vi "Read (Multiple Points).vi"(0 "VISA resource name":refnum<visa-resource-name>, 1 "Timeout (10000 ms)":i32=10000, 2 "Start Index (1)":i32=1, 3 "End Index(10)":i32=10, 5 "Buffer Name (\"\")":string, 7 "Capture Mode(0: Scan)":i32(ring) items=["Scan", "Trigger"], 9 "Clear Buffer (No)":bool, 11 "error in (no error)":errorcluster, 12 "Buffer Element1 ()":i32(ring) items=["", "Date", "Extra", "Formatted", "Fractional", "Reading", "Relative", "Seconds", "Status", "Time", "Tstamp", "Unit", "CHAN", "Extra Format", "Extra Unit"], 13 "Buffer Element2 ()":i32(ring) items=["", "Date", "Extra", "Formatted", "Fractional", "Reading", "Relative", "Seconds", "Status", "Time", "Tstamp", "Unit", "CHAN", "Extra Form", "Extra Unit"], 14 "Get Full Buffer":bool=TRUE) -> (4 "VISA resource name out":refnum<visa-resource-name>, 6 "Measurements":dbl[](array[numeric]), 15 "error out":errorcluster)   [LabVIEW 2020, in "Keithley DMM6500 DAQ6500 Series.lvlib"]
doc: "Reads and returns multiple measurements from the instrument. Use this VI when you want to take multiple measurements using an immediate trigger. Use the low-level VIs for other triggering options."
uses:
  <instrlib>/Keithley DMM6500 DAQ6500 Series/Keithley DMM6500 DAQ6500 Series.lvlib
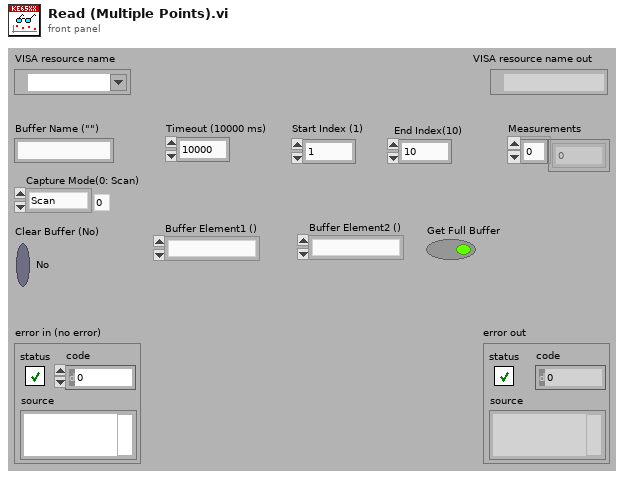
[diagram p1: front panel]
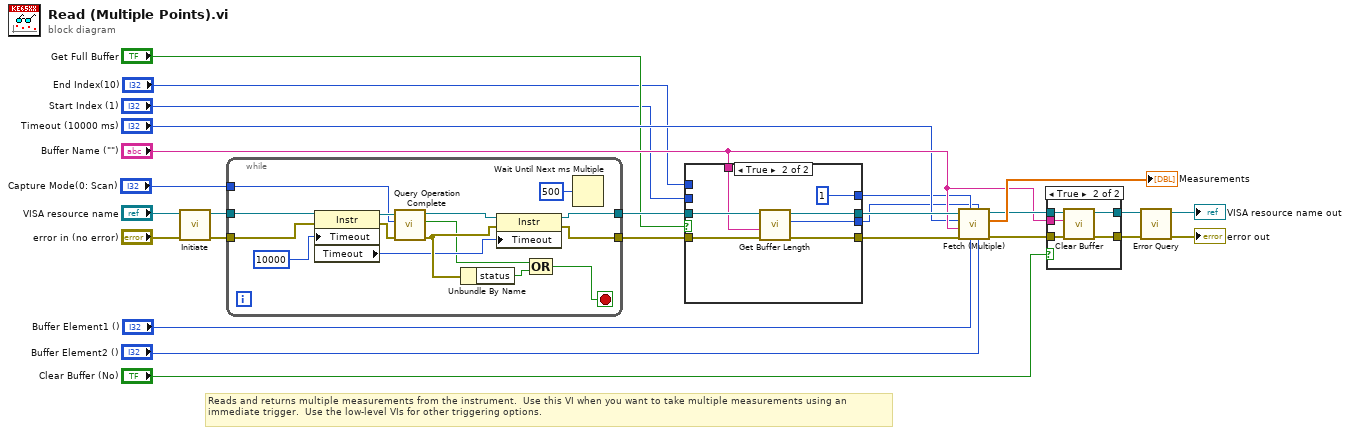
[diagram p0: block diagram]
diagram:
  # "Reads and returns multiple measurements from the instrument.  Use this VI when you want to take multiple measurements using an immediate trigger.  Use the low-level VIs for other triggering options."
  n1 = call <instrlib>:"Initiate.vi"("error in (no error)"="error in (no error)", "VISA resource name"="VISA resource name") -> ("error out"=w19:errorcluster, "VISA resource name out"=w20:refnum<visa-resource-name>)  [unwired: 8 in]
  n2 = while {
    tunnel: w20 -> [w38]
    tunnel: w19 -> [w37]
    tunnel: [w34] -> w16
    tunnel: [w33] -> w15
    tunnel: "Capture Mode(0: Scan)" -> [w27]
    stop <- w40 stop-if-true
    n3 = property on="Property Node" class="Instr"(reference=w38, error in=w37, "Timeout"=u32 10000 ("General Settings:Timeout Value")) -> (reference out=w36:refnum<visa-resource-name>, error out=w35:errorcluster, "Timeout"=w30:u32)
    n4 = call <instrlib>:"Query Operation Complete.vi"("error in (no error)"=w35, "Capture Mode (0: Scan)"=w27, "VISA resource name"=w36) -> ("error out"=w31:errorcluster, "Complete"=w28:bool, "VISA resource name out"=w32:refnum<visa-resource-name>)  [unwired: 6 in]
    n5 = Unbundle By Name(w31) -> ("status"=w39:bool)
    n6 = property on="Property Node" class="Instr"(reference=w32, error in=w31, "Timeout"=w30) -> (reference out=w34:refnum<visa-resource-name>, error out=w33:errorcluster)
    n7 = Compound Arithmetic op=OR(w28, w39) -> (w40:bool)
    n8 = Wait Until Next ms Multiple(millisecond multiple=u32 500) -> ()  [unwired: 1 out]
  }
  n9 = case shown="True" "Get Full Buffer" {
    tunnel: [w43 w52] -> w18
    tunnel: [w42 w51] -> w17
    tunnel: w16 -> [w43 w50]
    tunnel: w15 -> [w42 w49]
    tunnel: [w44 w48] -> w1
    tunnel: "Buffer Name (\"\")" -> [_ w47]
    tunnel: "Start Index (1)" -> [w45 _]
    tunnel: "End Index(10)" -> [w44 _]
    tunnel: [w45 1 ("Start Index (1)")] -> w2
    frame False {
    }
    frame True {
      n10 = call <instrlib>:"Get Buffer Length.vi"("error in (no error)"=w49, "Buffer Name ()"=w47, "VISA resource name"=w50) -> ("error out"=w51:errorcluster, "Buffer Count"=w48:i32, "VISA resource name out"=w52:refnum<visa-resource-name>)  [unwired: 6 in]
    }
  }
  n11 = call <instrlib>:"Fetch (Multiple).vi"("Buffer Element2 ()"="Buffer Element2 ()", "End Index (10)"=w1, "Buffer Element1 ()"="Buffer Element1 ()", "Start Index (1)"=w2, "error in (no error)"=w17, "Buffer Name (defbuffer1)"="Buffer Name (\"\")", "Timeout (100000 ms)"="Timeout (10000 ms)", "VISA resource name"=w18) -> ("error out"=w22:errorcluster, "Measurements"=→"Measurements":dbl[], "VISA resource name out"=w23:refnum<visa-resource-name>)  [unwired: 1 in]
  n12 = case shown="True" "Clear Buffer (No)" {
    tunnel: [w54 w59] -> w12
    tunnel: [w53 w58] -> w11
    tunnel: w23 -> [w54 w57]
    tunnel: w22 -> [w53 w56]
    tunnel: "Buffer Name (\"\")" -> [_ w55]
    frame False {
    }
    frame True {
      n13 = call <instrlib>:"Clear Buffer.vi"("error in (no error)"=w56, "Buffer Name (\"\")"=w55, "VISA resource name"=w57) -> ("error out"=w58:errorcluster, "VISA resource name out"=w59:refnum<visa-resource-name>)  [unwired: 7 in]
    }
  }
  n14 = call <instrlib>:"Error Query.vi"("error in (no error)"=w11, "VISA resource name"=w12) -> ("error out"=→"error out":errorcluster, "VISA resource name out"=→"VISA resource name out":refnum<visa-resource-name>)  [unwired: 6 in, 2 out]
